vi "Write Analogue.vi"(8 "error in (no error)":errorcluster, 10 "Outbput":bool, 11 "PS in":refnum<class "AIO.lvclass">) -> (0 "error out":errorcluster, 3 "PS out":refnum<class "AIO.lvclass">)   [LabVIEW 2021, in "HAL.lvlib" / "AIO.lvclass"]
uses:
  AIO.lvclass
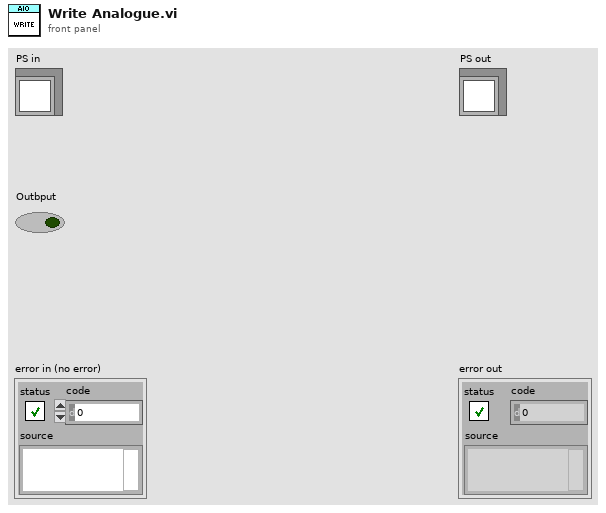
[diagram p1: front panel]
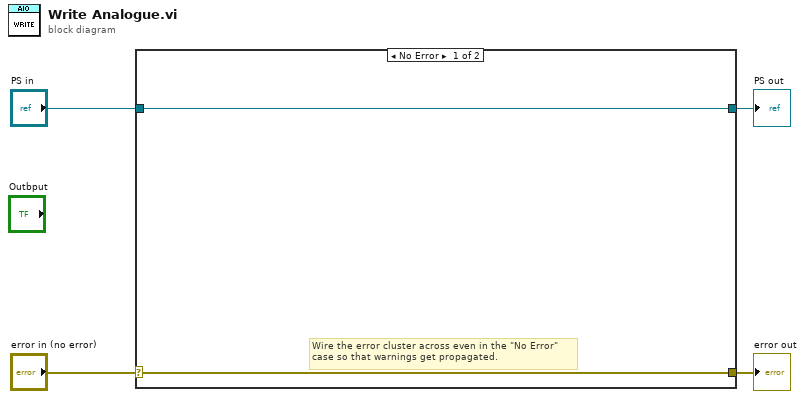
[diagram p0: block diagram]
diagram:
  n1 = case shown="No Error" "error in (no error)" {
    selector: "error in (no error)" -> [w5 w8]
    tunnel: [w5 w8] -> w3
    tunnel: [w6 w7] -> w1
    tunnel: "PS in" -> [w6 w7]
    frame No Error {
      # "Wire the error cluster across even in the \"No Error\"\ncase so that warnings get propagated."
    }
    frame Error {
    }
  }
  "error out" <- w3
  "PS out" <- w1
